vi "qpsk.vi"() -> ()   [LabVIEW 2014]
uses:
  <vilib>/Analysis/NI_AALPro.lvlib
panel:
  out "Waveform Chart":dbl[](graph)
  out "Array":bool[](array[boolean])
  out "Array":bool[](array[boolean])
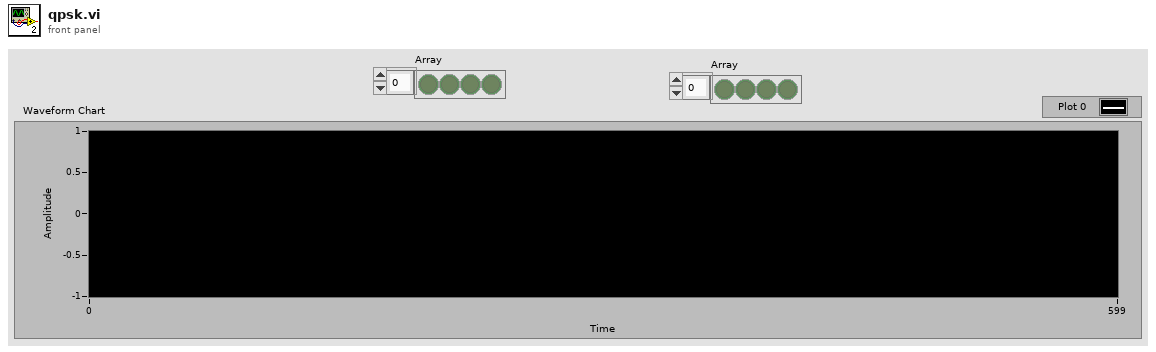
[diagram p1: front panel]
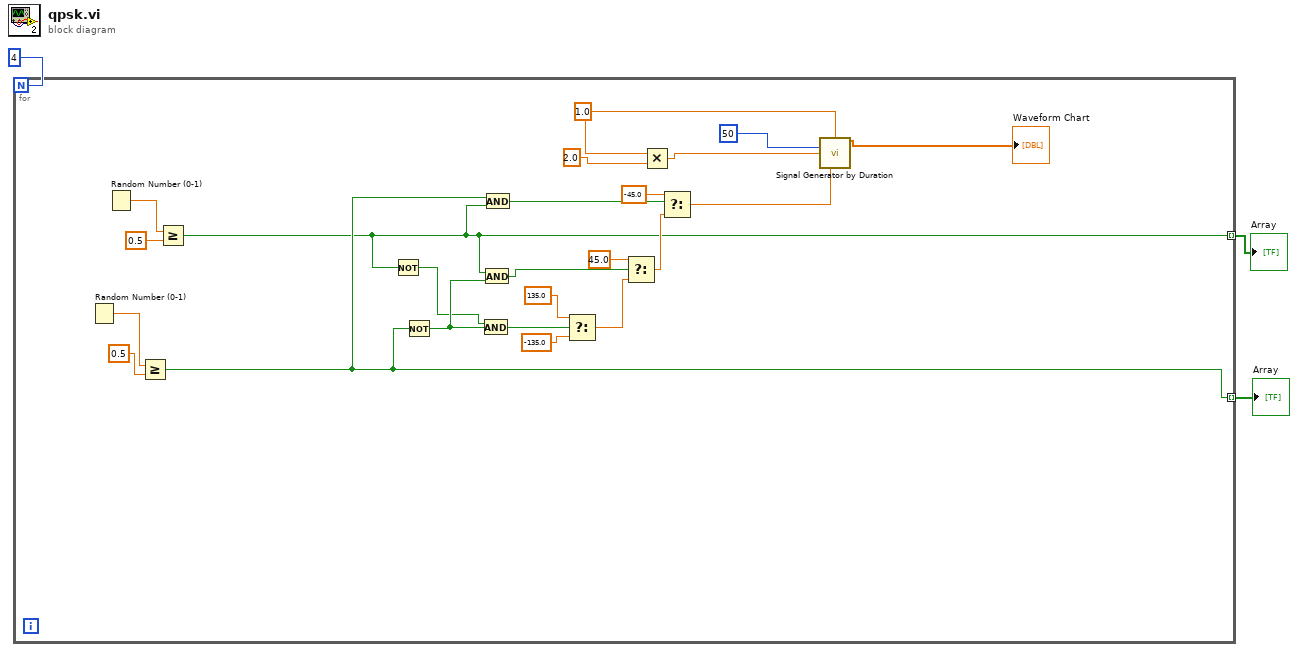
[diagram p0: block diagram]
diagram:
  n1 = for {
    N: 4 -> [_]
    tunnel: [w6] -> w2 mode=indexing
    tunnel: [w22] -> w1 mode=indexing
    w11 = 1.0 ("duration")
    n2 = Random Number (0-1)() -> (number: 0 to 1=w23:dbl)
    n3 = Random Number (0-1)() -> (number: 0 to 1=w25:dbl)
    n4 = Greater Or Equal?(x=w23, y=0.5) -> (x >= y?=w22:bool)
    n5 = Greater Or Equal?(x=w25, y=0.5) -> (x >= y?=w6:bool)
    n6 = Not(x=w6) -> (.not. x?=w5:bool)
    n7 = Not(x=w22) -> (.not. x?=w7:bool)
    n8 = And(x=w5, y=w7) -> (x .and. y?=w19:bool)
    n9 = And(x=w6, y=w7) -> (x .and. y?=w16:bool)
    n10 = And(x=w22, y=w6) -> (x .and. y?=w14:bool)
    n11 = Select(t=135.0, s=w19, f=-135.0) -> (s? t:f=w21:dbl)
    n12 = Select(t=45.0, s=w16, f=w21) -> (s? t:f=w20:dbl)
    n13 = Multiply(x=w11, y=2.0) -> (x*y=w8:dbl)
    n14 = Select(t=-45.0, s=w14, f=w20) -> (s? t:f=w12:dbl)
    n15 = call <vilib>:"Signal Generator by Duration.vi"("duration"=w11, "# of samples"=50, "frequency"=w8, "phase in"=w12) -> ("signal"=→"Waveform Chart":dbl[])  [unwired: 8 in, 3 out]
  }
  "Array" <- w2
  "Array" <- w1
